vi "read_pressure(SubVI).vi"() -> (0 "error out":errorcluster={"status"=FALSE, "code"=1073676294, "source"="VISA Read in datataker.vi"}, 1 "CC read error":errorcluster={"status"=FALSE, "code"=1073676294, "source"="VISA Read in datataker.vi"}, 2 "CC pressure (mbar)":string="2.4e", 3 "Array":dbl[](array[numeric]), 5 "Pirani pressure (mbar)":string)   [LabVIEW 2013]
uses:
  <vilib>/Instr/_visa.llb/VISA Configure Serial Port (Instr).vi
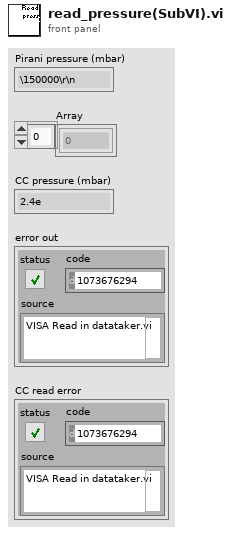
[diagram p1: front panel]
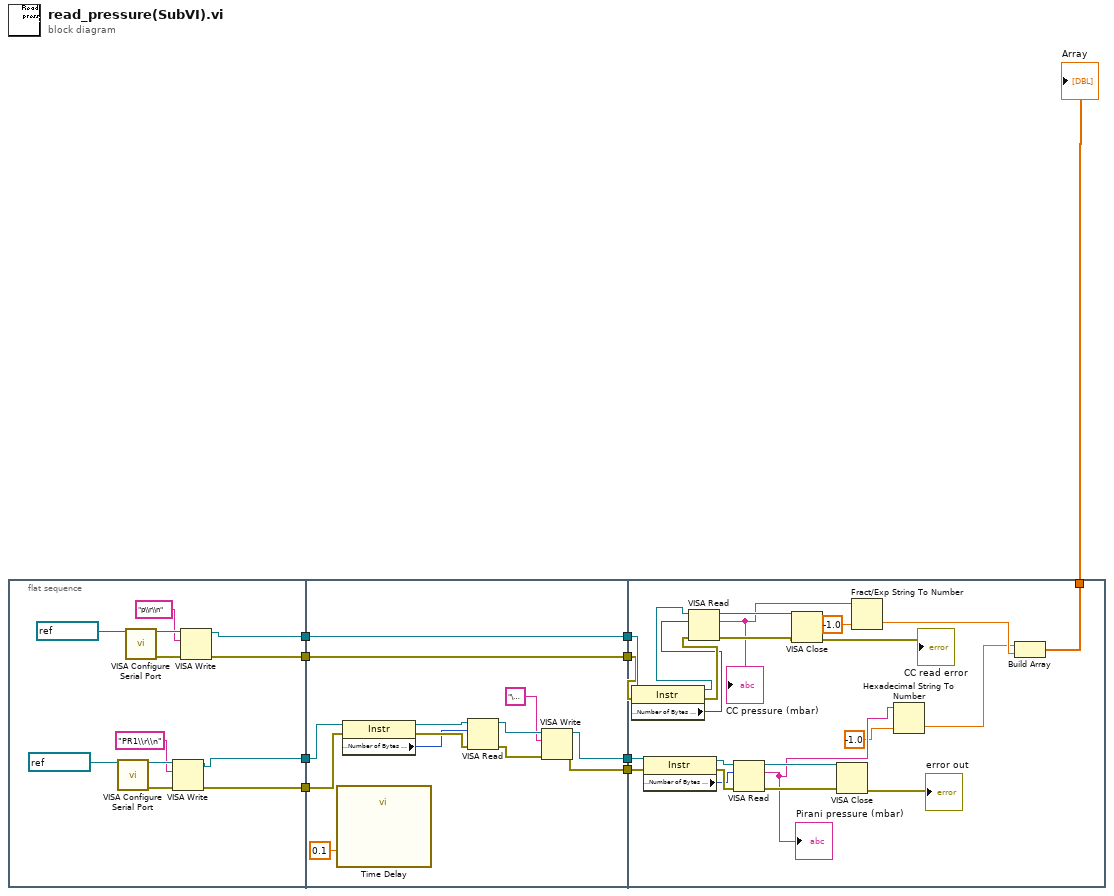
[diagram p0: block diagram]
diagram:
  n1 = flat-sequence {
    tunnel: [w17] -> w9
    tunnel: [w16] -> w8
    tunnel: [w11] -> w7
    tunnel: [w10] -> w6
    tunnel: [w25] -> w5
    tunnel: w9 -> [w31]
    tunnel: w8 -> [w30]
    tunnel: w7 -> [w33]
    tunnel: [w33] -> w4
    tunnel: w6 -> [w32]
    tunnel: [w32] -> w3
    tunnel: [w23] -> w2
    tunnel: w5 -> [w50]
    tunnel: w4 -> [w55]
    tunnel: w3 -> [w53]
    tunnel: w2 -> [w42]
    tunnel: [w39] -> w1
    frame #0 {
      n2 = call-poly "VISA Configure Serial Port"("VISA resource name"=refnum<visa-resource-name> "COM3") -> ("VISA resource name out"=w20:refnum<visa-resource-name>, "error out"=w18:errorcluster)  [unwired: 8 in, 5 out]
      n3 = call-poly "VISA Configure Serial Port"("VISA resource name"=refnum<visa-resource-name> "COM5") -> ("VISA resource name out"=w14:refnum<visa-resource-name>, "error out"=w12:errorcluster)  [unwired: 8 in, 5 out]
      n4 = VISA Write(VISA resource name=w20, write buffer="PR1\\r\\n", error in (no error)=w18) -> (VISA resource name out=w17:refnum<visa-resource-name>, error out=w16:errorcluster)  [unwired: 1 out]
      n5 = VISA Write(VISA resource name=w14, write buffer="p\\r\\n", error in (no error)=w12) -> (VISA resource name out=w11:refnum<visa-resource-name>, error out=w10:errorcluster)  [unwired: 1 out]
    }
    frame #1 {
      n6 = call "Time Delay"("Delay Time (s)"=0.1) -> ()  [unwired: 10 in, 1 out]
      n7 = property class="Instr"(reference=w31, error in=w30) -> (reference out=w28:refnum<visa-resource-name>, error out=w29:errorcluster, "Serial Settings:Number of Bytes at Serial Port"=w27:u32)
      n8 = VISA Read(VISA resource name=w28, byte count=w27, error in (no error)=w29) -> (VISA resource name out=w26:refnum<visa-resource-name>, error out=w24:errorcluster)  [unwired: 2 out]
      n9 = VISA Write(VISA resource name=w26, write buffer="\u0005", error in (no error)=w24) -> (VISA resource name out=w25:refnum<visa-resource-name>, error out=w23:errorcluster)  [unwired: 1 out]
    }
    frame #2 {
      n10 = property class="Instr"(reference=w55, error in=w53) -> (reference out=w54:refnum<visa-resource-name>, error out=w52:errorcluster, "Serial Settings:Number of Bytes at Serial Port"=w51:u32)
      n11 = property class="Instr"(reference=w50, error in=w42) -> (reference out=w49:refnum<visa-resource-name>, error out=w48:errorcluster, "Serial Settings:Number of Bytes at Serial Port"=w43:u32)
      n12 = VISA Read(VISA resource name=w54, byte count=w51, error in (no error)=w52) -> (VISA resource name out=w56:refnum<visa-resource-name>, read buffer=w41:string, error out=w47:errorcluster)  [unwired: 1 out]
      "CC pressure (mbar)" <- w41
      n13 = VISA Read(VISA resource name=w49, byte count=w43, error in (no error)=w48) -> (VISA resource name out=w57:refnum<visa-resource-name>, read buffer=w37:string, error out=w45:errorcluster)  [unwired: 1 out]
      "Pirani pressure (mbar)" <- w37
      n14 = VISA Close(VISA resource name=w56, error in (no error)=w47) -> (error out=→"CC read error":errorcluster)
      n15 = VISA Close(VISA resource name=w57, error in (no error)=w45) -> (error out=→"error out":errorcluster)
      n16 = Fract/Exp String To Number(string=w41, default (0 dbl)=-1.0 ("default (0 DBL)")) -> (number=w40:dbl)  [unwired: 2 in, 1 out]
      n17 = Hexadecimal String To Number(string=w37, default (0uL)=-1.0 ("default (0 DBL)")) -> (number=w35:dbl)  [unwired: 1 in, 1 out]
      n18 = Build Array(w35, w40) -> (w39:dbl[])
    }
  }
  "Array" <- w1
